vi "Example Threshold.vi"() -> ()   [LabVIEW 2010]
uses:
  C:/tf/play/labview/Tinkerforge.dll
  Tinkerforge.dll
panel:
  in  "stop":bool
  out "callback counter":i32
  out "last temperature (°C)":sgl
  in  "uid":string="dHd"
  in  "port":i32=4223
  in  "host":string="localhost"
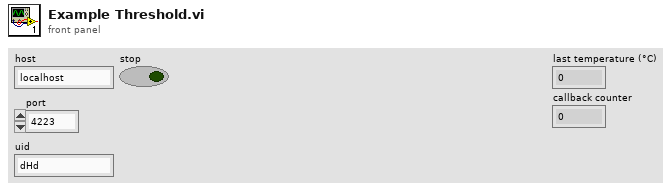
[diagram p1: front panel]
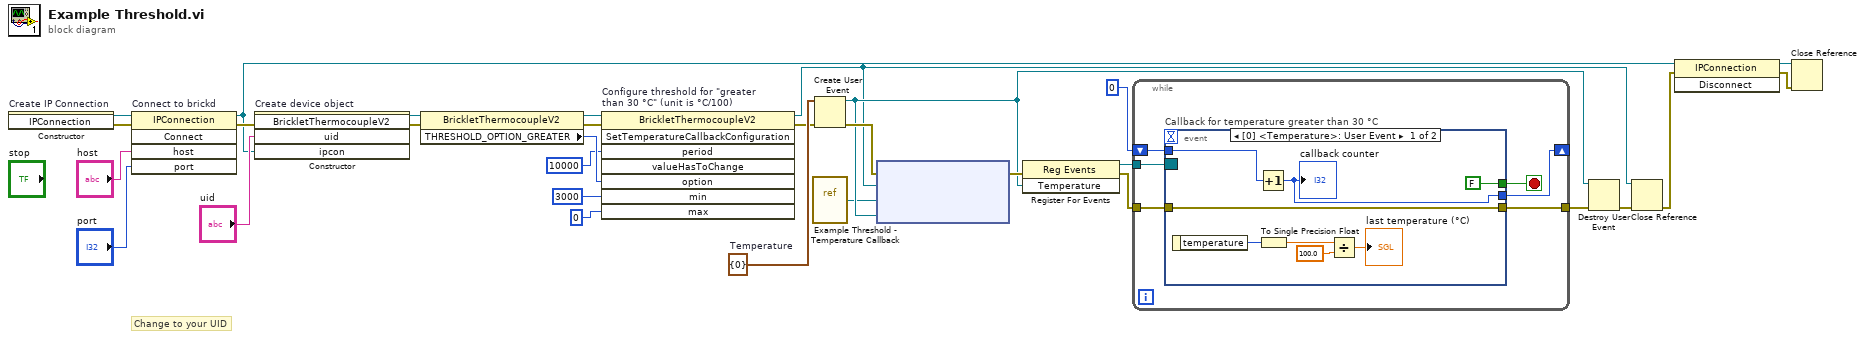
[diagram p0: block diagram]
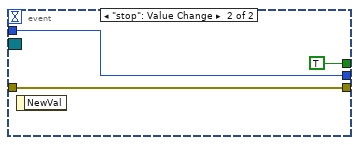
[diagram p2: hidden frame]
diagram:
  w14 = cluster{"temperature":i32} {"temperature"=0}  # Temperature
  # "Change to your UID"
  n1 = constructor on="Create IP Connection" class="IPConnection"() -> (reference out=w30:refnum<k24>, error out=w8:errorcluster)  [unwired: 3 in, 1 out]
  n2 = invoke on="Connect to brickd" class="IPConnection" method="Connect"(reference=w30, error in=w8, "host"="host", "port"="port") -> (reference out=w23:refnum<k24>, error out=w26:errorcluster)  [unwired: 1 in, 3 out]
  n3 = constructor on="Create device object" class="BrickletThermocoupleV2"(error in=w26, "uid"="uid", "ipcon"=w23) -> (reference out=w7:refnum<k24>, error out=w6:errorcluster)  [unwired: 2 in, 3 out]
  n4 = property class="BrickletThermocoupleV2"(reference=w7, error in=w6) -> (reference out=w10:refnum<k24>, error out=w11:errorcluster, "THRESHOLD_OPTION_GREATER"=w3:u16)
  n5 = invoke on="Configure threshold for \"greater\nthan 30 °C\" (unit is °C/100)" class="BrickletThermocoupleV2" method="SetTemperatureCallbackConfiguration"(reference=w10, error in=w11, "period"=i64 10000, "option"=w3, "min"=3000, "max"=0) -> (reference out=w13:refnum<k24>, error out=w12:errorcluster)  [unwired: 2 in, 6 out]
  n6 = vi-ref "Example Threshold - Temperature Callback.vi"() -> ("vi reference"=w1:refnum<vi>)
  n7 = Create User Event(user event datatype=w14, error in=w12) -> (user event=w16:refnum<user-event>, error out=w21:errorcluster)
  n8 = node ("Register Event Callback")(w21, w13, w1, w16) -> (w20:errorcluster)  [unwired: 1 in, 1 out]
  n9 = register-events(error in=w20, w16) -> (reference out=w19:refnum<event-registration>, error out=w17:errorcluster)  [unwired: 1 in]
  n10 = while {
    tunnel: w19 -> [w36]
    tunnel: [w35] -> w18
    tunnel: w17 -> [w34]
    shift-right: [w32] -> _
    shift-left: 0 -> [w33]
    stop <- w31 stop-if-true
    n11 = event "Callback for temperature greater than 30 °C" shown="[0] <Temperature>: User Event" {
      selector: w36 -> [_ _]
      dyn-events: _ -> [_ _]
      timeout: _ -> [_ _]
      tunnel: [w41 w45] -> w35
      tunnel: w34 -> [w41 w45]
      tunnel: w33 -> [w39 w46]
      tunnel: [w38 w46] -> w32
      tunnel: [FALSE TRUE] -> w31
      event User Event {
        n12 = event-data() -> ("temperature"=w42:i32)  [unwired: 1 in]
        n13 = Increment(x=w39) -> (x+1=w38:i32)
        "callback counter" <- w38
        n14 = To Single Precision Float(number=w42) -> (single precision float=w43:sgl)
        n15 = Divide(x=w43, y=sgl 100.0) -> (x/y=→"last temperature (°C)":sgl)
      }
      event "stop": Value Change {
        n16 = event-data() -> ()  [unwired: 1 in, 1 out]
      }
    }
  }
  n17 = Destroy User Event(user event=w16, error in=w18) -> (error out=w15:errorcluster)
  n18 = Close Reference(reference=w13, error in (no error)=w15) -> (error out=w25:errorcluster)
  n19 = invoke class="IPConnection" method="Disconnect"(reference=w23, error in=w25) -> (reference out=w22:refnum<k24>, error out=w24:errorcluster)  [unwired: 1 in, 1 out]
  n20 = Close Reference(reference=w22, error in (no error)=w24) -> ()  [unwired: 1 out]
